vi "FdxCmdRxUDPCreatePortCvi.vi"(8 "error in":errorcluster, 9 "UdpDescription":T1 {"PortType" items=["FDX_UDP_SAMPLING", "FDX_UDP_QUEUING", "FDX_UDP_RX_SAP", "FDX_UDP_TX_SAP"]}, 11 "InstrumentHandle_port":u32) -> (0 "error out":errorcluster, 1 "UdpHandle":u32, 3 "InstrumentHandle_port":u32)   [LabVIEW 2020, in "AIM664LV.lvlib"]
doc: "This function creates a port to receive data from a specified UDP connection oriented port. This function can be used only if the receiver is not running. This function assumes that AiFdxCmdRxVLControl was previously called in order to enable a VL for reception. On this VL this function creates an FDX communication Rx-port."
uses:
  AIM664LV.lvlib
  AFDX_LibraryAdmin/FdxGlobalDllPath.vi
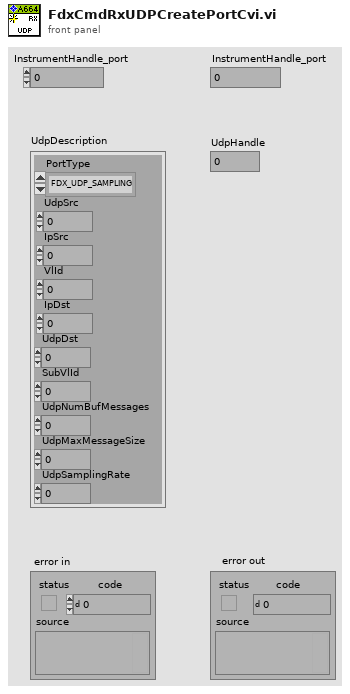
[diagram p1: front panel]
types:
  T1 = cluster{"PortType":u32, "UdpSrc":u32, "IpSrc":u32, "VlId":u32, "IpDst":u32, "UdpDst":u32, "SubVlId":u32, "UdpNumBufMessages":u32, "UdpMaxMessageSize":u32, "UdpSamplingRate":u32}
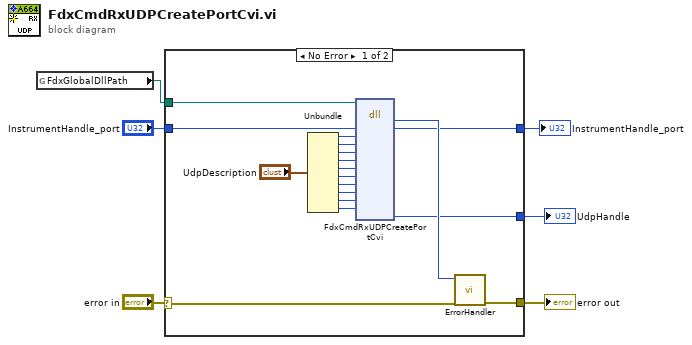
[diagram p0: block diagram]
diagram:
  n1 = global read "FdxGlobalDllPath.vi" "FdxGlobalDllPath"() -> (w4:path)
  n2 = case shown="No Error" "error in" {
    selector: "error in" -> [w23 w26]
    tunnel: [w24 w26] -> w6
    tunnel: w4 -> [w10 _]
    tunnel: "InstrumentHandle_port" -> [w9 w25]
    tunnel: [w8 w25] -> w2
    tunnel: [w7 _] -> w1
    frame No Error {
      n3 = Unbundle("UdpDescription") -> ("PortType"=w20:u32, "UdpSrc"=w19:u32, "IpSrc"=w18:u32, "VlId"=w17:u32, "IpDst"=w16:u32, "UdpDst"=w15:u32, "SubVlId"=w14:u32, "UdpNumBufMessages"=w13:u32, "UdpMaxMessageSize"=w12:u32, "UdpSamplingRate"=w11:u32)
      n4 = dll-call lib="aim_fdx.19.dll" fn="FdxCmdRxUDPCreatePortCvi"(path in=w10, "InstrumentHandle"=w9, "PortType"=w20, "UdpSrc"=w19, "IpSrc"=w18, "VlId"=w17, "IpDst"=w16, "UdpDst"=w15, "SubVlId"=w14, "UdpNumBufMessages"=w13, "UdpMaxMessageSize"=w12, "UdpSamplingRate"=w11) -> ("status"=w22:i32, "InstrumentHandle"=w8:u32, "UdpHandle"=w7:u32)  [unwired: 12 in, 3 out]
      n5 = call "ErrorHandler.vi"("error in"=w23, "AIM Error"=w22) -> ("error out"=w24:errorcluster)  [unwired: 9 in]
    }
    frame Error {
    }
  }
  "error out" <- w6
  "InstrumentHandle_port" <- w2
  "UdpHandle" <- w1
